vi "S7_Extract_Data_TCP.vi"(11 "Data Recieved":u8[](array[numeric])) -> (0 "Error":u16, 1 "PDU Exchanged":bool, 2 "Data Valid":bool, 3 "Data":u8[](array[numeric]))   [LabVIEW 2018, in "S7 TCP.lvlib"]
uses:
  S7 TCP.lvlib
panel:
  out "Length in Bytes":u16
  out "Data Transport Size":u8
  out "Returning Write Data":bool
  out "Number of Items Read":u8
  out "Returning Read Data":bool
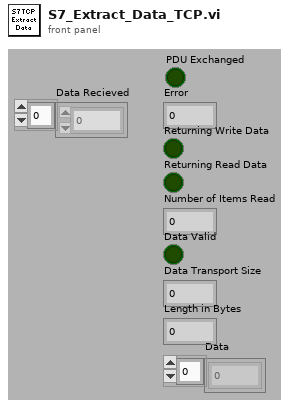
[diagram p1: front panel]
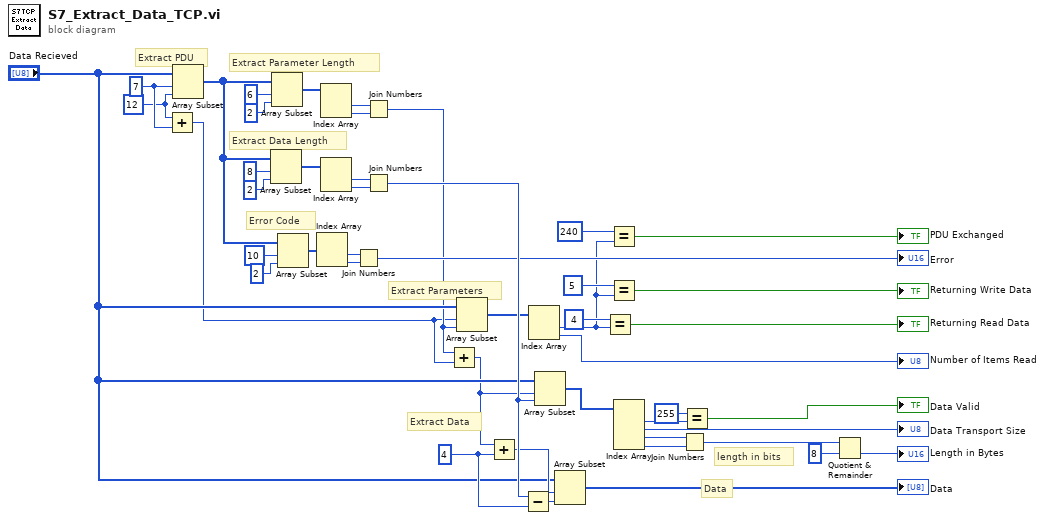
[diagram p0: block diagram]
diagram:
  w47 = 4 ("y")
  w2 = 12 ("length")
  w3 = 7 ("index")
  # "Error Code"
  # "Data"
  # "length in bits"
  # "Extract Parameters"
  # "Extract Data"
  # "Extract Data Length"
  # "Extract Parameter Length"
  # "Extract PDU"
  n1 = Add(x=w2, y=w3) -> (x+y=w1:i32)
  n2 = Array Subset(array="Data Recieved", index=w3, length=w2) -> (w17:u8[])
  n3 = Array Subset(array=w17, index=8, length=2) -> (w23:u8[])
  n4 = Array Subset(array=w17, index=6, length=2) -> (w18:u8[])
  n5 = Array Subset(array=w17, index=10, length=2) -> (w39:u8[])
  n6 = Index Array(array=w39) -> (element #1=w36:u8, element #2=w40:u8)  [unwired: 2 in]
  n7 = Index Array(array=w18) -> (element #1=w19:u8, element #2=w20:u8)  [unwired: 2 in]
  n8 = Index Array(array=w23) -> (element #1=w22:u8, element #2=w21:u8)  [unwired: 2 in]
  n9 = Join Numbers(hi=w36, lo=w40) -> ((hi.lo)=→"Error":u16)
  n10 = Join Numbers(hi=w19, lo=w20) -> ((hi.lo)=w24:u16)
  n11 = Join Numbers(hi=w22, lo=w21) -> ((hi.lo)=w46:u16)
  n12 = Add(x=w24, y=w1) -> (x+y=w41:i32)
  n13 = Array Subset(array="Data Recieved", index=w1, length=w24) -> (w25:u8[])
  n14 = Add(x=w41, y=w47) -> (x+y=w44:i32)
  n15 = Subtract(x=w46, y=w47) -> (x-y=w45:i32)
  n16 = Index Array(array=w25) -> (element #1=w5:u8, element #2=→"Number of Items Read":u8)  [unwired: 2 in]
  n17 = Array Subset(array="Data Recieved", index=w41, length=w46) -> (w42:u8[])
  n18 = Array Subset(array="Data Recieved", index=w44, length=w45) -> (→"Data":u8[])
  n19 = Equal?(x=u8 4, y=w5) -> (x = y?=→"Returning Read Data":bool)
  n20 = Equal?(x=u8 240, y=w5) -> (x = y?=→"PDU Exchanged":bool)
  n21 = Equal?(x=u8 5, y=w5) -> (x = y?=→"Returning Write Data":bool)
  n22 = Index Array(array=w42) -> (element #1=w31:u8, element #2=→"Data Transport Size":u8, element #3=w33:u8, element #4=w34:u8)  [unwired: 4 in]
  n23 = Join Numbers(hi=w33, lo=w34) -> ((hi.lo)=w10:u16)
  n24 = Equal?(x=u8 255, y=w31) -> (x = y?=→"Data Valid":bool)
  n25 = Quotient & Remainder(x=w10, y=u16 8) -> (floor(x/y)=→"Length in Bytes":u16)  [unwired: 1 out]
